vi "CaseRegister1.vi"() -> ()   [LabVIEW 2021]
panel:
  out "String":string
  in  "Numeric":dbl
  out "Waveform Chart":dbl(graph)
  in  "Set Point":dbl(slide) scale=0.0..20.0
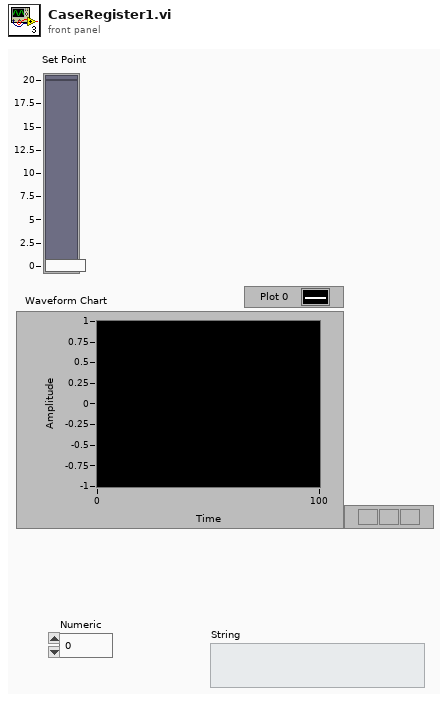
[diagram p1: front panel]
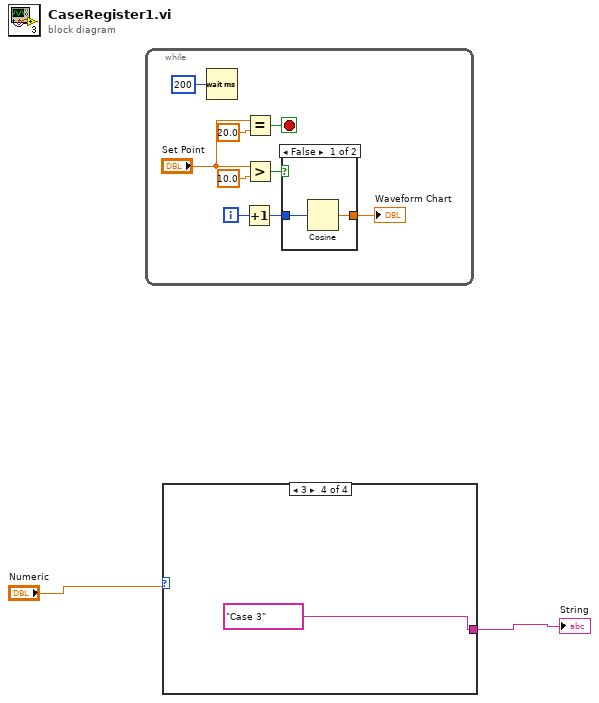
[diagram p0: block diagram]
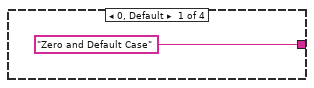
[diagram p2: hidden frame]
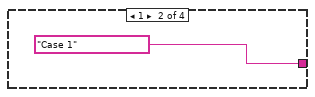
[diagram p3: hidden frame]
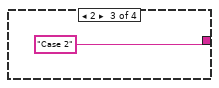
[diagram p4: hidden frame]
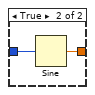
[diagram p5: hidden frame]
diagram:
  n1 = while {
    i -> [w9]
    stop <- w5 stop-if-true
    n2 = Wait (ms)(milliseconds to wait=u32 200) -> ()  [unwired: 1 out]
    n3 = Increment(x=w9) -> (x+1=w8:i32)
    n4 = Equal?(x="Set Point", y=20.0) -> (x = y?=w5:bool)
    n5 = Greater?(x="Set Point", y=10.0) -> (0:w10:bool)
    n6 = case shown="False" w10 {
      tunnel: w8 -> [w13 w15]
      tunnel: [w12 w14] -> w7
      frame False {
        n7 = Cosine(x=w13) -> (cos(x)=w12:dbl)
      }
      frame True {
        n8 = Sine(x=w15) -> (sin(x)=w14:dbl)
      }
    }
    "Waveform Chart" <- w7
  }
  n9 = case shown="3" "Numeric" {
    tunnel: ["Zero and Default Case" "Case 1" "Case 2" "Case 3"] -> w1
    frame 0, Default {
    }
    frame 1 {
    }
    frame 2 {
    }
    frame 3 {
    }
  }
  "String" <- w1
